vi "MSTAutoSummarySpecial.vi"() -> ()   [LabVIEW 2012]
uses:
  <vilib>/Utility/NIReport.llb/NI_report.lvclass
  <vilib>/addons/database/Connection.llb/DB Tools Open Connec (Path).vi
  <vilib>/addons/database/Connection.llb/Conn Execute.vi
  <vilib>/addons/database/Recordset.llb/Rec Fetch Recordset Data (R).vi
  <vilib>/addons/database/Recordset.llb/Rec Destroy - Connection.vi
  <vilib>/Utility/NIReport.llb/Append Text Table to Report (wrap).vi
  <vilib>/addons/database/_DB Variant To Data/Database Variant To Data.xnode
  <vilib>/addons/database/NI_Database_API.lvlib
  <vilib>/Utility/NIReport.llb/Excel/NI_Excel.lvclass
  <vilib>/addons/_office/NI_ReportGenerationToolkit.lvlib
panel:
  in  "Report Template":path=path "O:/Monitor/Report/MSTDailyReport.xls"
  in  "Table Control":string[][](table)
  in  "Table Control 2":string[][](table)
  out "error out 4":errorcluster
  out "error out 3":errorcluster
  out "appended array 3":string[](array[string])
  out "recordset data 3":variant[][](array[variant])
  out "error out":errorcluster
  out "appended array":string[](array[string])
  out "recordset data":variant[][](array[variant])
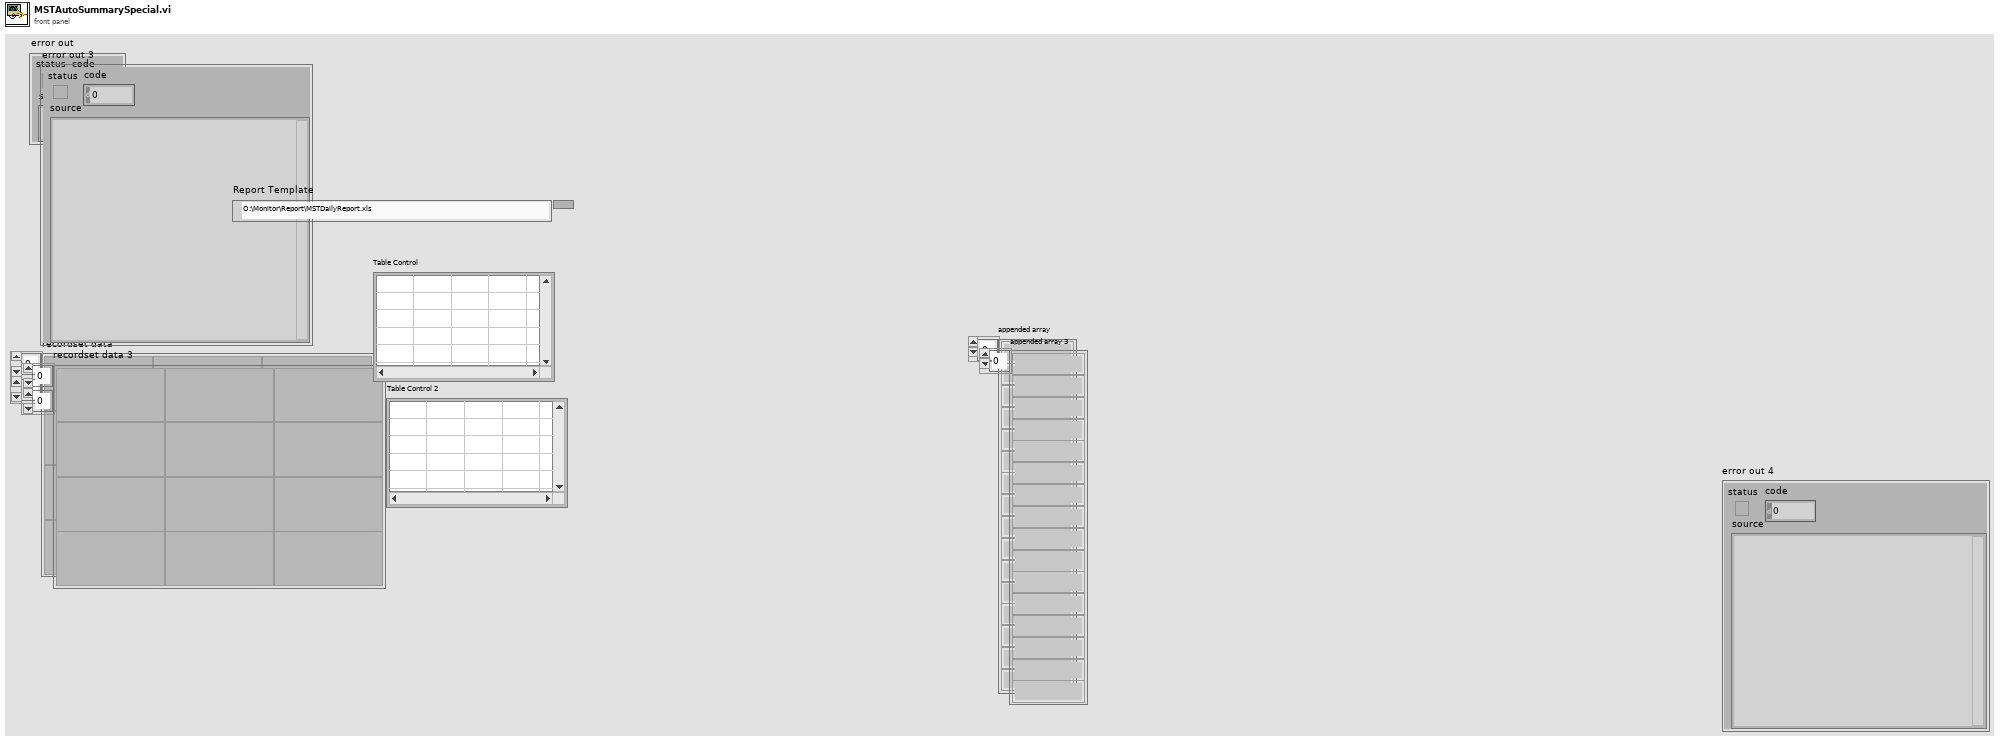
[diagram p1: front panel]
types:
  T1 = typedef "NI_Database_API.lvlib/Conn ObjectReference.ctl" = refnum<k1>
  T2 = typedef "NI_Database_API.lvlib/Rec ObjectReference.ctl" = refnum<k1>
  T3 = enum16{"Standard Report", "HTML", "Word", "Excel"}
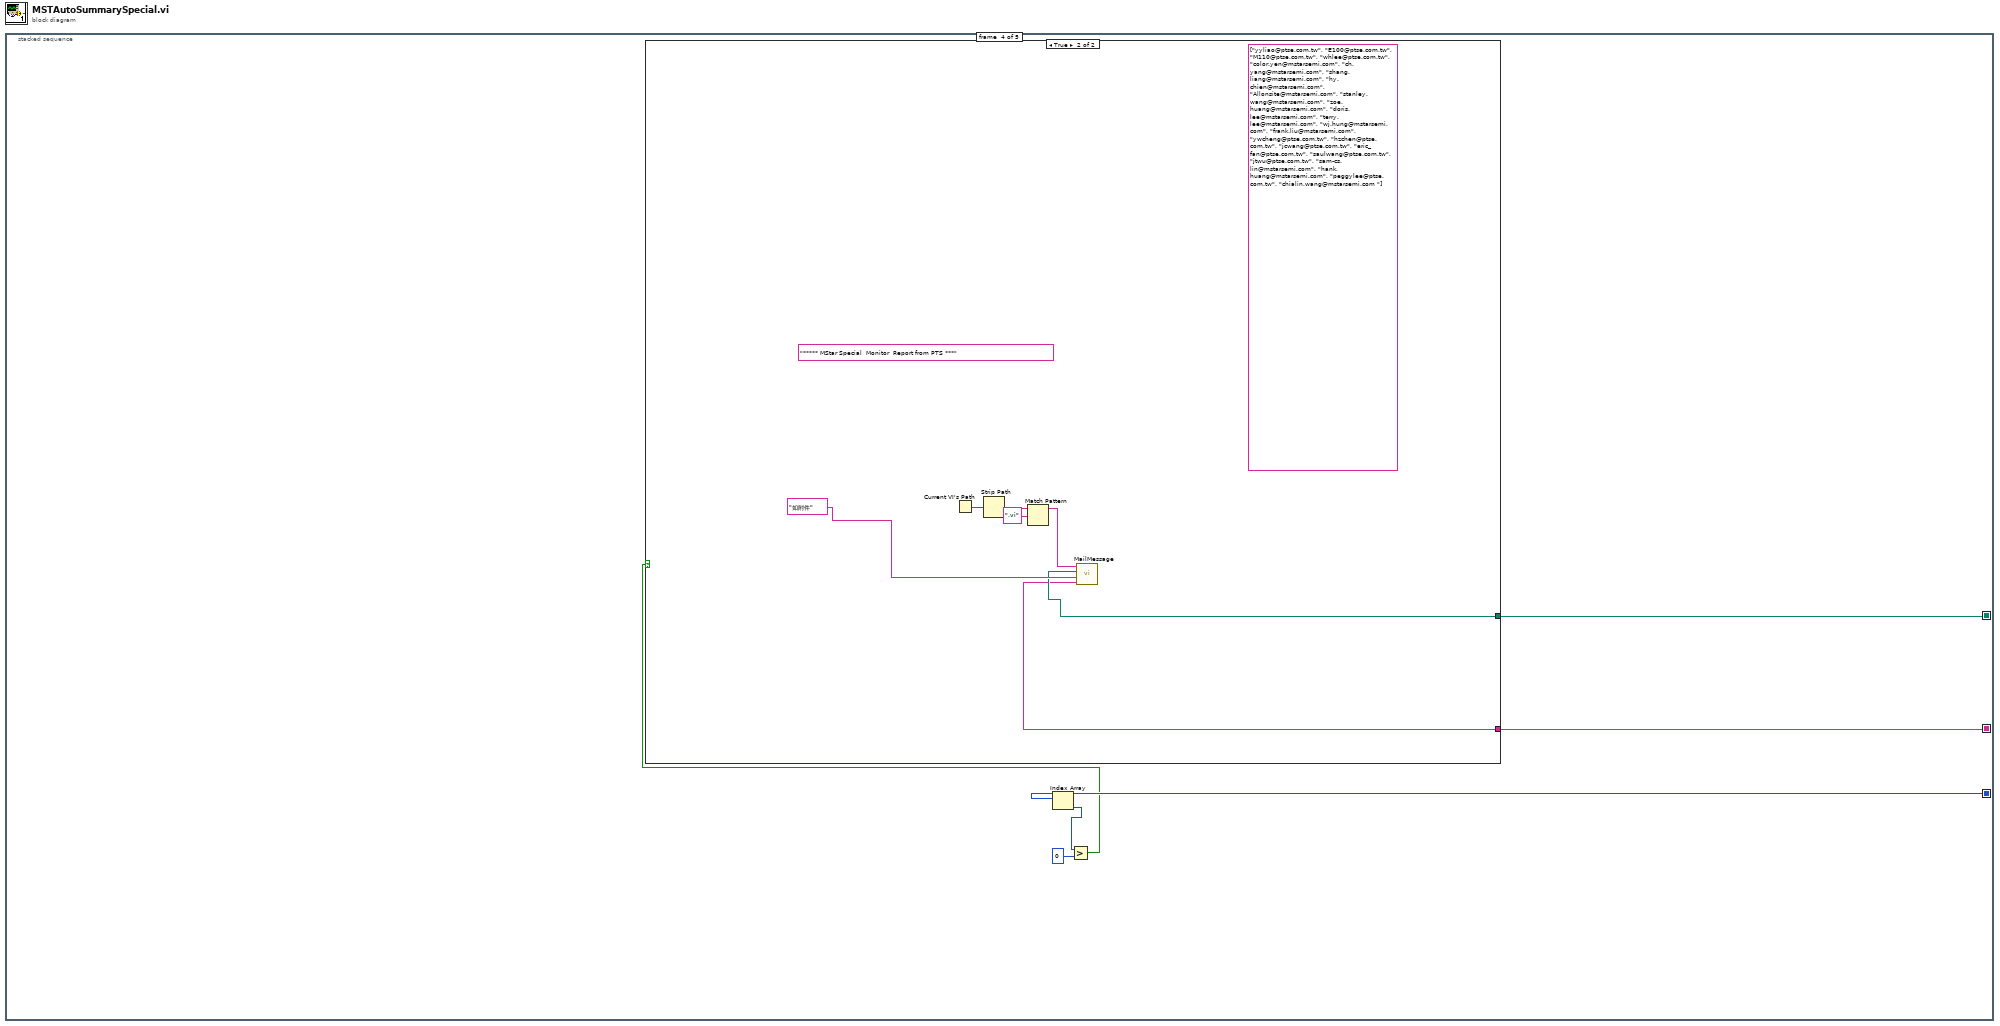
[diagram p0: block diagram]
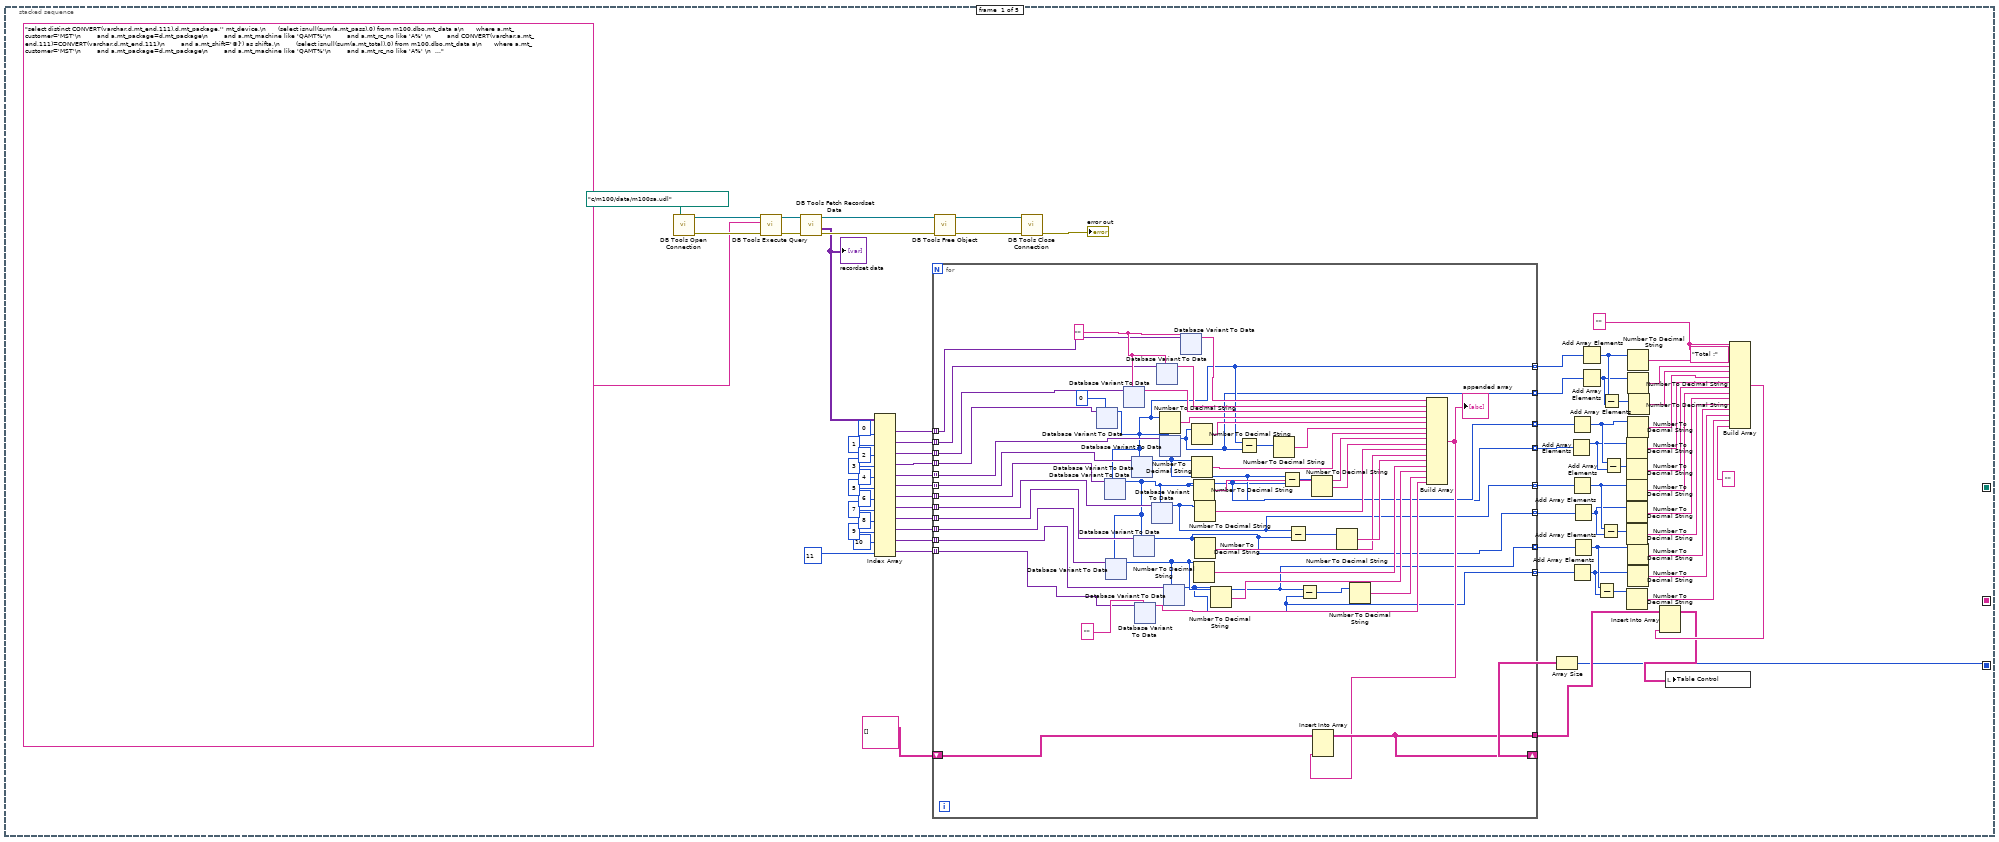
[diagram p2: hidden frame]
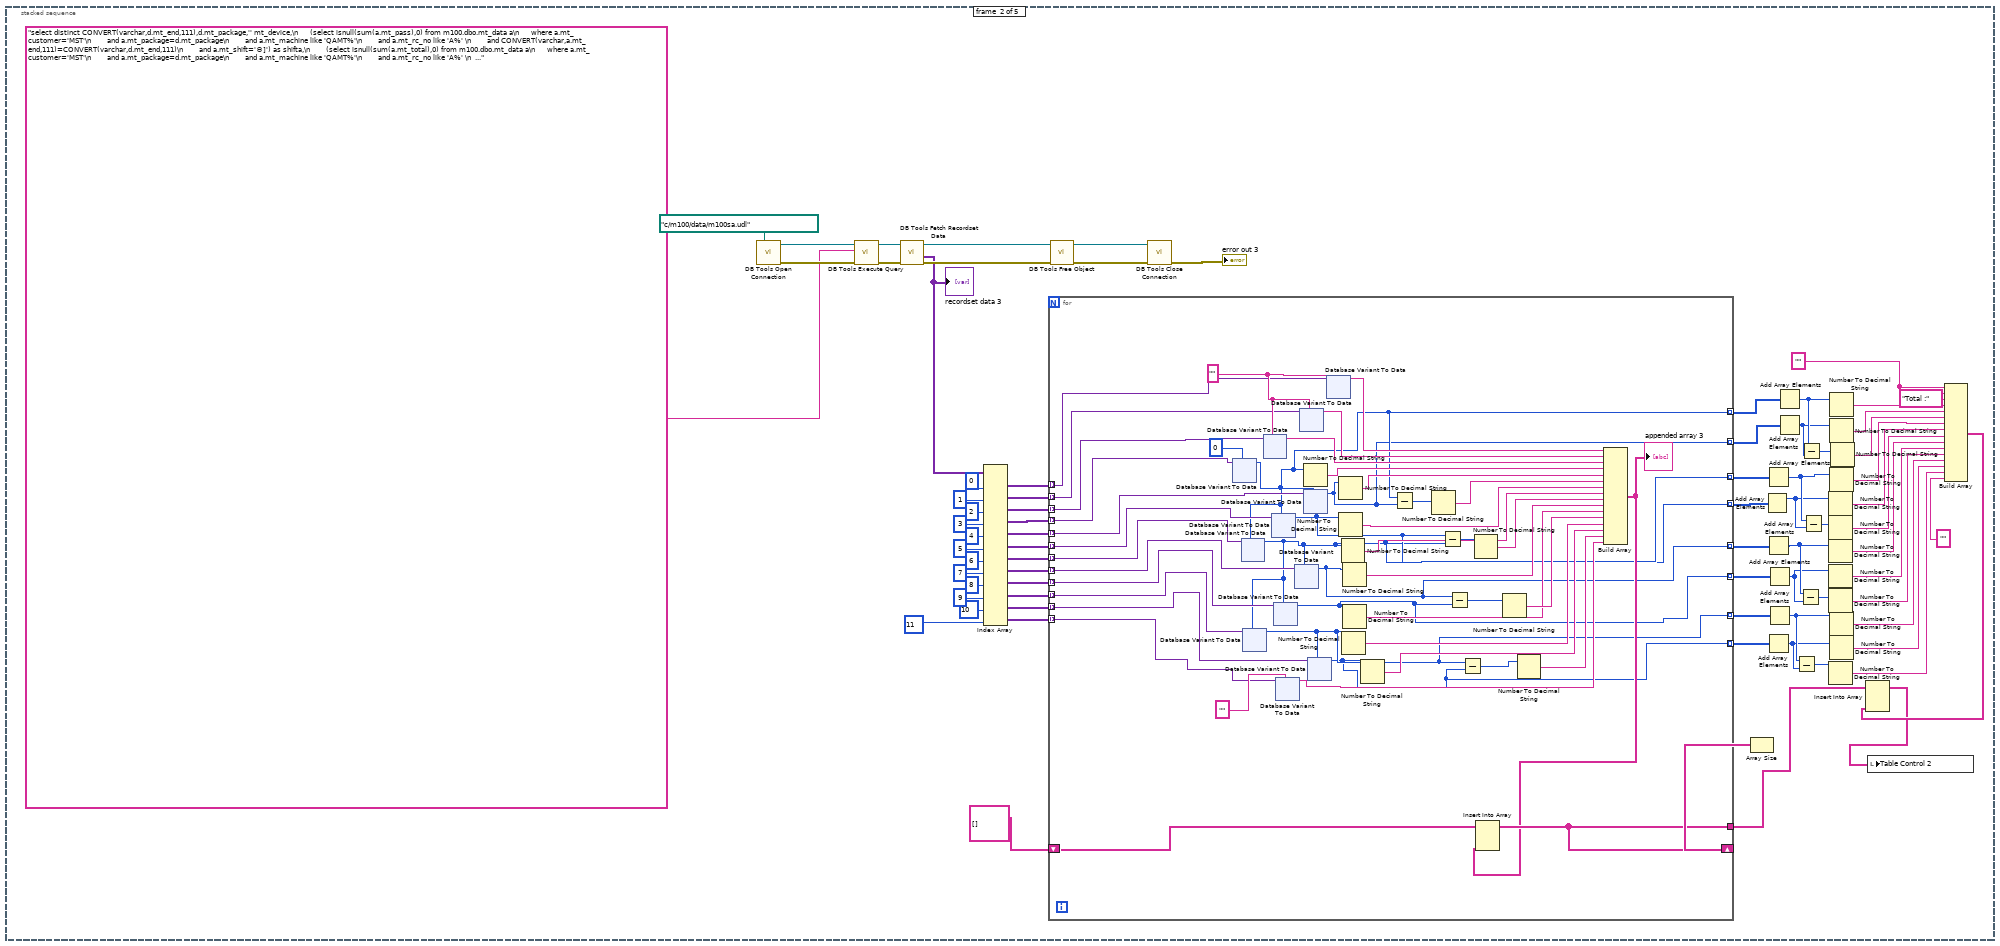
[diagram p3: hidden frame]
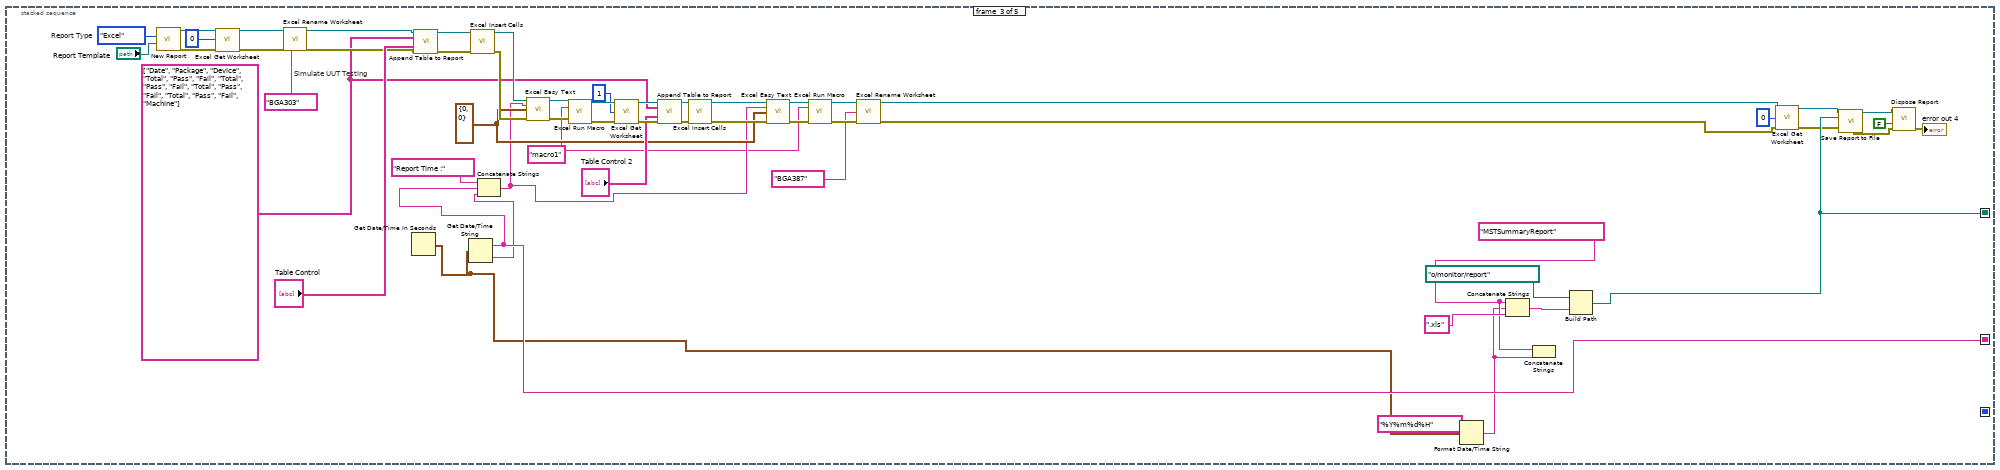
[diagram p4: hidden frame]
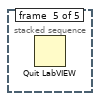
[diagram p6: hidden frame]
diagram:
  n1 = stacked-sequence {
    seq-local: [_ _ w1055 _ _] -> [_ _ _ w1075 _]
    seq-local: [_ _ w1054 _ _] -> [_ _ _ w1074 _]
    seq-local: [w1 _ _ _ _] -> [_ _ _ w1073 _]
    frame #0 {
      w37 = ""
      n2 = call-poly <vilib>:"DB Tools Open Connection.vi"("connection information"=path "c:/m100/data/m100sa.udl") -> ("error out"=w72:errorcluster, "connection reference"=w76:T1)  [unwired: 7 in]
      n3 = call-poly <vilib>:"DB Tools Execute Query.vi"("error in (no error)"=w72, "SQL query"="select distinct CONVERT(varchar,d.mt_end,111),d.mt_package,'' mt_device,\n      (select isnull(sum(a.mt_pass),0) from m100.dbo.mt_data a\n      where a.mt_customer='MST'\n        and a.mt_package=d.mt_package\n        and a.mt_machine like 'QAMT%'\n        and a.mt_rc_no like 'A%' \n        and CONVERT(varchar,a.mt_end,111)=CONVERT(varchar,d.mt_end,111)\n        and a.mt_shift='©]') as shifta,\n        (select isnull(sum(a.mt_total),0) from m100.dbo.mt_data a\n      where a.mt_customer='MST'\n        and a.mt_package=d.mt_package\n        and a.mt_machine like 'QAMT%'\n        and a.mt_rc_no like 'A%' \n        and CONVERT(varchar,a.mt_end,111)=CONVERT(varchar,d.mt_end,111)\n        and a.mt_shift='©]') as shifta1,\n        (select isnull(sum(b.mt_pass),0) from m100.dbo.mt_data b\n      where b.mt_customer='MST'\n        and b.mt_package=d.mt_package\n        and b.mt_machine like 'QAMT%'\n        and b.mt_rc_no like 'A%' \n        and CONVERT(varchar,b.mt_end,111)=CONVERT(varchar,d.mt_end,111)\n        and b.mt_shift='¦­') as shiftb,\n        (select isnull(sum(b.mt_total),0) from m100.dbo.mt_data b\n      where b.mt_customer='MST'\n        and b.mt_package=d.mt_package\n        and b.mt_machine like 'QAMT%'\n        and b.mt_rc_no like 'A%' \n        and CONVERT(varchar,b.mt_end,111)=CONVERT(varchar,d.mt_end,111)\n        and b.mt_shift='¦­') as shiftb1,\n        (select isnull(sum(c.mt_pass),0) from m100.dbo.mt_data c\n      where c.mt_customer='MST'\n        and c.mt_package=d.mt_package\n        and c.mt_machine like 'QAMT%'\n        and c.mt_rc_no like 'A%' \n        and CONVERT(varchar,c.mt_end,111)=CONVERT(varchar,d.mt_end,111)\n        and c.mt_shift='¤¤') as shiftc,\n        (select isnull(sum(c.mt_total),0) from m100.dbo.mt_data c\n      where c.mt_customer='MST'\n        and c.mt_package=d.mt_package\n        and c.mt_machine like 'QAMT%'\n        and c.mt_rc_no like 'A%' \n        and CONVERT(varchar,c.mt_end,111)=CONVERT(varchar,d.mt_end,111)\n        and c.mt_shift='¤¤') as shiftc1,\n        SUM(mt_pass),SUM(mt_total),master.dbo.GetEntityNameFromDateToDateByPackage('MST',d.mt_package,CONVERT(varchar,d.mt_end,111),CONVERT(varchar,d.mt_end,111))\n  FROM [m100].[dbo].[mt_data] d\n  WHERE d.mt_customer='MST'\n    and d.mt_machine like 'QAMT%'\n    and d.mt_package like '%BGA303%'\n    AND CONVERT(varchar,d.mt_end,111) >= convert(varchar,getdate()-30,111)\n    AND CONVERT(varchar,d.mt_end,111) >= '2016/03/30'\n    and d.mt_pass > 0 and d.mt_rc_no like 'A%'\n      group by CONVERT(varchar,d.mt_end,111),d.mt_package", "connection reference"=w76) -> ("error out"=w71:errorcluster, "recordset reference"=w75:T2)  [unwired: 5 in]
      n4 = call-poly <vilib>:"DB Tools Fetch Recordset Data.vi"("error in (no error)"=w71, "recordset reference"=w75) -> ("error out"=w70:errorcluster, "recordset data"=w40:variant[][], "recordset reference out"=w74:T2)  [unwired: 3 in]
      "recordset data" <- w40
      n5 = Index Array(array=w40, index (col) #1=0 ("index (row)"), index (col) #2=1 ("index (col)"), index (col) #3=2 ("disabled index (col)"), index (col) #4=3 ("index (col)"), index (col) #5=4 ("index (col)"), index (col) #6=5 ("index (col)"), index (col) #7=6 ("index (col)"), index (col) #8=7 ("index (col)"), index (col) #9=8 ("index (col)"), index (col) #10=9 ("index (col)"), index (col) #11=10 ("index (col)"), index (col) #12=11 ("index (col)")) -> (element #1=w44:variant[], element #2=w43:variant[], element #3=w57:variant[], element #4=w56:variant[], element #5=w55:variant[], element #6=w54:variant[], element #7=w53:variant[], element #8=w52:variant[], element #9=w51:variant[], element #10=w50:variant[], element #11=w49:variant[], element #12=w48:variant[])  [unwired: 12 in]
      n6 = for {
        tunnel: w57 -> [w96] mode=indexing
        tunnel: w56 -> [w95] mode=indexing
        tunnel: w55 -> [w94] mode=indexing
        tunnel: w54 -> [w93] mode=indexing
        tunnel: w53 -> [w92] mode=indexing
        tunnel: w52 -> [w91] mode=indexing
        tunnel: w51 -> [w90] mode=indexing
        tunnel: w50 -> [w89] mode=indexing
        tunnel: w49 -> [w88] mode=indexing
        tunnel: w48 -> [w87] mode=indexing
        tunnel: [w123] -> w30
        shift-right: [w123] -> w46
        shift-left: string[][] [] ("array") -> [w122]
        tunnel: w44 -> [w98] mode=indexing
        tunnel: w43 -> [w97] mode=indexing
        tunnel: [w85] -> w39 mode=indexing
        tunnel: [w84] -> w38 mode=indexing
        tunnel: [w83] -> w28 mode=indexing
        tunnel: [w82] -> w27 mode=indexing
        tunnel: [w81] -> w18 mode=indexing
        tunnel: [w80] -> w17 mode=indexing
        tunnel: [w79] -> w10 mode=indexing
        tunnel: [w78] -> w9 mode=indexing
        w121 = ""
        n7 = xnode "Database Variant To Data"("database variant"=w95, "type"=0) -> ("data"=w85:i32)  [unwired: 1 in, 1 out]
        n8 = xnode "Database Variant To Data"("database variant"=w92, "type"=w85) -> ("data"=w82:i32)  [unwired: 1 in, 1 out]
        n9 = xnode "Database Variant To Data"("database variant"=w89, "type"=w82) -> ("data"=w79:i32)  [unwired: 1 in, 1 out]
        n10 = xnode "Database Variant To Data"("database variant"=w96, "type"=w121) -> ("data"=w104:string)  [unwired: 1 in, 1 out]
        n11 = xnode "Database Variant To Data"("database variant"=w93, "type"=w85) -> ("data"=w83:i32)  [unwired: 1 in, 1 out]
        n12 = xnode "Database Variant To Data"("database variant"=w90, "type"=w82) -> ("data"=w80:i32)  [unwired: 1 in, 1 out]
        n13 = xnode "Database Variant To Data"("database variant"=w87, "type"="") -> ("data"=w116:string)  [unwired: 1 in, 1 out]
        n14 = xnode "Database Variant To Data"("database variant"=w91, "type"=w82) -> ("data"=w81:i32)  [unwired: 1 in, 1 out]
        n15 = xnode "Database Variant To Data"("database variant"=w97, "type"=w121) -> ("data"=w101:string)  [unwired: 1 in, 1 out]
        n16 = Number To Decimal String(number=w85) -> (decimal integer string=w103:string)  [unwired: 1 in]
        n17 = xnode "Database Variant To Data"("database variant"=w94, "type"=w85) -> ("data"=w84:i32)  [unwired: 1 in, 1 out]
        n18 = xnode "Database Variant To Data"("database variant"=w88, "type"=w79) -> ("data"=w78:i32)  [unwired: 1 in, 1 out]
        n19 = xnode "Database Variant To Data"("database variant"=w98, "type"=w121) -> ("data"=w105:string)  [unwired: 1 in, 1 out]
        n20 = Number To Decimal String(number=w84) -> (decimal integer string=w102:string)  [unwired: 1 in]
        n21 = Number To Decimal String(number=w83) -> (decimal integer string=w119:string)  [unwired: 1 in]
        n22 = Number To Decimal String(number=w82) -> (decimal integer string=w118:string)  [unwired: 1 in]
        n23 = Number To Decimal String(number=w79) -> (decimal integer string=w112:string)  [unwired: 1 in]
        n24 = Number To Decimal String(number=w81) -> (decimal integer string=w108:string)  [unwired: 1 in]
        n25 = Number To Decimal String(number=w80) -> (decimal integer string=w109:string)  [unwired: 1 in]
        n26 = Number To Decimal String(number=w78) -> (decimal integer string=w113:string)  [unwired: 1 in]
        n27 = Subtract(x=w85, y=w84) -> (x-y=w100:i32)
        n28 = Number To Decimal String(number=w100) -> (decimal integer string=w99:string)  [unwired: 1 in]
        n29 = Subtract(x=w83, y=w82) -> (x-y=w107:i32)
        n30 = Subtract(x=w81, y=w80) -> (x-y=w111:i32)
        n31 = Subtract(x=w79, y=w78) -> (x-y=w115:i32)
        n32 = Number To Decimal String(number=w107) -> (decimal integer string=w106:string)  [unwired: 1 in]
        n33 = Number To Decimal String(number=w111) -> (decimal integer string=w110:string)  [unwired: 1 in]
        n34 = Number To Decimal String(number=w115) -> (decimal integer string=w114:string)  [unwired: 1 in]
        n35 = Build Array(w105, w101, w104, w103, w102, w99, w119, w118, w106, w108, w109, w110, w112, w113, w114, w116) -> (w86:string[])
        "appended array" <- w86
        n36 = Insert Into Array(array=w122, new element=w86) -> (w123:string[][])  [unwired: 2 in]
      }
      n37 = call-poly <vilib>:"DB Tools Free Object.vi"("error in (no error)"=w70, "recordset reference"=w74) -> ("error out"=w69:errorcluster, "connection reference"=w73:T1)  [unwired: 8 in]
      n38 = call <vilib>:"DB Tools Close Connection.vi"("error in (no error)"=w69, "connection reference"=w73) -> ("error out"=→"error out":errorcluster)  [unwired: 5 in]
      n39 = Array Size(array=w46) -> (size(s)=w1:i32[])
      n40 = Add Array Elements(numeric array=w27) -> (sum=w21:i32)
      n41 = Add Array Elements(numeric array=w28) -> (sum=w22:i32)
      n42 = Add Array Elements(numeric array=w18) -> (sum=w14:i32)
      n43 = Add Array Elements(numeric array=w9) -> (sum=w7:i32)
      n44 = Add Array Elements(numeric array=w17) -> (sum=w13:i32)
      n45 = Add Array Elements(numeric array=w10) -> (sum=w8:i32)
      n46 = Add Array Elements(numeric array=w39) -> (sum=w34:i32)
      n47 = Add Array Elements(numeric array=w38) -> (sum=w33:i32)
      n48 = Subtract(x=w8, y=w7) -> (x-y=w6:i32)
      n49 = Subtract(x=w14, y=w13) -> (x-y=w11:i32)
      n50 = Subtract(x=w34, y=w33) -> (x-y=w26:i32)
      n51 = Subtract(x=w22, y=w21) -> (x-y=w19:i32)
      n52 = Number To Decimal String(number=w21) -> (decimal integer string=w23:string)  [unwired: 1 in]
      n53 = Number To Decimal String(number=w19) -> (decimal integer string=w20:string)  [unwired: 1 in]
      n54 = Number To Decimal String(number=w14) -> (decimal integer string=w16:string)  [unwired: 1 in]
      n55 = Number To Decimal String(number=w13) -> (decimal integer string=w15:string)  [unwired: 1 in]
      n56 = Number To Decimal String(number=w11) -> (decimal integer string=w12:string)  [unwired: 1 in]
      n57 = Number To Decimal String(number=w6) -> (decimal integer string=w3:string)  [unwired: 1 in]
      n58 = Number To Decimal String(number=w34) -> (decimal integer string=w36:string)  [unwired: 1 in]
      n59 = Number To Decimal String(number=w33) -> (decimal integer string=w35:string)  [unwired: 1 in]
      n60 = Number To Decimal String(number=w22) -> (decimal integer string=w25:string)  [unwired: 1 in]
      n61 = Number To Decimal String(number=w8) -> (decimal integer string=w5:string)  [unwired: 1 in]
      n62 = Number To Decimal String(number=w7) -> (decimal integer string=w4:string)  [unwired: 1 in]
      n63 = Number To Decimal String(number=w26) -> (decimal integer string=w32:string)  [unwired: 1 in]
      n64 = Build Array(w37, w37, "Total :" ("element"), w36, w35, w32, w25, w23, w20, w16, w15, w12, w5, w4, w3, "") -> (w31:string[])
      n65 = Insert Into Array(array=w30, new element=w31) -> (w29:string[][])  [unwired: 2 in]
      n66 = local write "Table Control"(w29) -> ()
    }
    frame #1 {
      w543 = ""
      n67 = call-poly <vilib>:"DB Tools Open Connection.vi"("connection information"=path "c:/m100/data/m100sa.udl") -> ("error out"=w578:errorcluster, "connection reference"=w582:T1)  [unwired: 7 in]
      n68 = call-poly <vilib>:"DB Tools Execute Query.vi"("error in (no error)"=w578, "SQL query"="select distinct CONVERT(varchar,d.mt_end,111),d.mt_package,'' mt_device,\n      (select isnull(sum(a.mt_pass),0) from m100.dbo.mt_data a\n      where a.mt_customer='MST'\n        and a.mt_package=d.mt_package\n        and a.mt_machine like 'QAMT%'\n        and a.mt_rc_no like 'A%' \n        and CONVERT(varchar,a.mt_end,111)=CONVERT(varchar,d.mt_end,111)\n        and a.mt_shift='©]') as shifta,\n        (select isnull(sum(a.mt_total),0) from m100.dbo.mt_data a\n      where a.mt_customer='MST'\n        and a.mt_package=d.mt_package\n        and a.mt_machine like 'QAMT%'\n        and a.mt_rc_no like 'A%' \n        and CONVERT(varchar,a.mt_end,111)=CONVERT(varchar,d.mt_end,111)\n        and a.mt_shift='©]') as shifta1,\n        (select isnull(sum(b.mt_pass),0) from m100.dbo.mt_data b\n      where b.mt_customer='MST'\n        and b.mt_package=d.mt_package\n        and b.mt_machine like 'QAMT%'\n        and b.mt_rc_no like 'A%' \n        and CONVERT(varchar,b.mt_end,111)=CONVERT(varchar,d.mt_end,111)\n        and b.mt_shift='¦­') as shiftb,\n        (select isnull(sum(b.mt_total),0) from m100.dbo.mt_data b\n      where b.mt_customer='MST'\n        and b.mt_package=d.mt_package\n        and b.mt_machine like 'QAMT%'\n        and b.mt_rc_no like 'A%' \n        and CONVERT(varchar,b.mt_end,111)=CONVERT(varchar,d.mt_end,111)\n        and b.mt_shift='¦­') as shiftb1,\n        (select isnull(sum(c.mt_pass),0) from m100.dbo.mt_data c\n      where c.mt_customer='MST'\n        and c.mt_package=d.mt_package\n        and c.mt_machine like 'QAMT%'\n        and c.mt_rc_no like 'A%' \n        and CONVERT(varchar,c.mt_end,111)=CONVERT(varchar,d.mt_end,111)\n        and c.mt_shift='¤¤') as shiftc,\n        (select isnull(sum(c.mt_total),0) from m100.dbo.mt_data c\n      where c.mt_customer='MST'\n        and c.mt_package=d.mt_package\n        and c.mt_machine like 'QAMT%'\n        and c.mt_rc_no like 'A%' \n        and CONVERT(varchar,c.mt_end,111)=CONVERT(varchar,d.mt_end,111)\n        and c.mt_shift='¤¤') as shiftc1,\n        SUM(mt_pass),SUM(mt_total),master.dbo.GetEntityNameFromDateToDateByPackage('MST',d.mt_package,CONVERT(varchar,d.mt_end,111),CONVERT(varchar,d.mt_end,111))\n  FROM [m100].[dbo].[mt_data] d\n  WHERE d.mt_customer='MST'\n    and d.mt_machine like 'QAMT%'\n    and d.mt_package like '%BGA387%'\n    AND CONVERT(varchar,d.mt_end,111) >= convert(varchar,getdate()-30,111)\n    AND CONVERT(varchar,d.mt_end,111) >= '2016/03/30'\n    and d.mt_pass > 0 and d.mt_rc_no like 'A%'\n      group by CONVERT(varchar,d.mt_end,111),d.mt_package", "connection reference"=w582) -> ("error out"=w577:errorcluster, "recordset reference"=w581:T2)  [unwired: 5 in]
      n69 = call-poly <vilib>:"DB Tools Fetch Recordset Data.vi"("error in (no error)"=w577, "recordset reference"=w581) -> ("error out"=w576:errorcluster, "recordset data"=w546:variant[][], "recordset reference out"=w580:T2)  [unwired: 3 in]
      "recordset data 3" <- w546
      n70 = Index Array(array=w546, index (col) #1=0 ("index (row)"), index (col) #2=1 ("index (col)"), index (col) #3=2 ("disabled index (col)"), index (col) #4=3 ("index (col)"), index (col) #5=4 ("index (col)"), index (col) #6=5 ("index (col)"), index (col) #7=6 ("index (col)"), index (col) #8=7 ("index (col)"), index (col) #9=8 ("index (col)"), index (col) #10=9 ("index (col)"), index (col) #11=10 ("index (col)"), index (col) #12=11 ("index (col)")) -> (element #1=w550:variant[], element #2=w549:variant[], element #3=w563:variant[], element #4=w562:variant[], element #5=w561:variant[], element #6=w560:variant[], element #7=w559:variant[], element #8=w558:variant[], element #9=w557:variant[], element #10=w556:variant[], element #11=w555:variant[], element #12=w554:variant[])  [unwired: 12 in]
      n71 = for {
        tunnel: w563 -> [w602] mode=indexing
        tunnel: w562 -> [w601] mode=indexing
        tunnel: w561 -> [w600] mode=indexing
        tunnel: w560 -> [w599] mode=indexing
        tunnel: w559 -> [w598] mode=indexing
        tunnel: w558 -> [w597] mode=indexing
        tunnel: w557 -> [w596] mode=indexing
        tunnel: w556 -> [w595] mode=indexing
        tunnel: w555 -> [w594] mode=indexing
        tunnel: w554 -> [w593] mode=indexing
        tunnel: [w629] -> w536
        shift-right: [w629] -> w552
        shift-left: string[][] [] ("array") -> [w628]
        tunnel: w550 -> [w604] mode=indexing
        tunnel: w549 -> [w603] mode=indexing
        tunnel: [w591] -> w545 mode=indexing
        tunnel: [w590] -> w544 mode=indexing
        tunnel: [w589] -> w534 mode=indexing
        tunnel: [w588] -> w533 mode=indexing
        tunnel: [w587] -> w524 mode=indexing
        tunnel: [w586] -> w523 mode=indexing
        tunnel: [w585] -> w516 mode=indexing
        tunnel: [w584] -> w515 mode=indexing
        w627 = ""
        n72 = xnode "Database Variant To Data"("database variant"=w601, "type"=0) -> ("data"=w591:i32)  [unwired: 1 in, 1 out]
        n73 = xnode "Database Variant To Data"("database variant"=w598, "type"=w591) -> ("data"=w588:i32)  [unwired: 1 in, 1 out]
        n74 = xnode "Database Variant To Data"("database variant"=w595, "type"=w588) -> ("data"=w585:i32)  [unwired: 1 in, 1 out]
        n75 = xnode "Database Variant To Data"("database variant"=w602, "type"=w627) -> ("data"=w610:string)  [unwired: 1 in, 1 out]
        n76 = xnode "Database Variant To Data"("database variant"=w599, "type"=w591) -> ("data"=w589:i32)  [unwired: 1 in, 1 out]
        n77 = xnode "Database Variant To Data"("database variant"=w596, "type"=w588) -> ("data"=w586:i32)  [unwired: 1 in, 1 out]
        n78 = xnode "Database Variant To Data"("database variant"=w593, "type"="") -> ("data"=w622:string)  [unwired: 1 in, 1 out]
        n79 = xnode "Database Variant To Data"("database variant"=w597, "type"=w588) -> ("data"=w587:i32)  [unwired: 1 in, 1 out]
        n80 = xnode "Database Variant To Data"("database variant"=w603, "type"=w627) -> ("data"=w607:string)  [unwired: 1 in, 1 out]
        n81 = Number To Decimal String(number=w591) -> (decimal integer string=w609:string)  [unwired: 1 in]
        n82 = xnode "Database Variant To Data"("database variant"=w600, "type"=w591) -> ("data"=w590:i32)  [unwired: 1 in, 1 out]
        n83 = xnode "Database Variant To Data"("database variant"=w594, "type"=w585) -> ("data"=w584:i32)  [unwired: 1 in, 1 out]
        n84 = xnode "Database Variant To Data"("database variant"=w604, "type"=w627) -> ("data"=w611:string)  [unwired: 1 in, 1 out]
        n85 = Number To Decimal String(number=w590) -> (decimal integer string=w608:string)  [unwired: 1 in]
        n86 = Number To Decimal String(number=w589) -> (decimal integer string=w625:string)  [unwired: 1 in]
        n87 = Number To Decimal String(number=w588) -> (decimal integer string=w624:string)  [unwired: 1 in]
        n88 = Number To Decimal String(number=w585) -> (decimal integer string=w618:string)  [unwired: 1 in]
        n89 = Number To Decimal String(number=w587) -> (decimal integer string=w614:string)  [unwired: 1 in]
        n90 = Number To Decimal String(number=w586) -> (decimal integer string=w615:string)  [unwired: 1 in]
        n91 = Number To Decimal String(number=w584) -> (decimal integer string=w619:string)  [unwired: 1 in]
        n92 = Subtract(x=w591, y=w590) -> (x-y=w606:i32)
        n93 = Number To Decimal String(number=w606) -> (decimal integer string=w605:string)  [unwired: 1 in]
        n94 = Subtract(x=w589, y=w588) -> (x-y=w613:i32)
        n95 = Subtract(x=w587, y=w586) -> (x-y=w617:i32)
        n96 = Subtract(x=w585, y=w584) -> (x-y=w621:i32)
        n97 = Number To Decimal String(number=w613) -> (decimal integer string=w612:string)  [unwired: 1 in]
        n98 = Number To Decimal String(number=w617) -> (decimal integer string=w616:string)  [unwired: 1 in]
        n99 = Number To Decimal String(number=w621) -> (decimal integer string=w620:string)  [unwired: 1 in]
        n100 = Build Array(w611, w607, w610, w609, w608, w605, w625, w624, w612, w614, w615, w616, w618, w619, w620, w622) -> (w592:string[])
        "appended array 3" <- w592
        n101 = Insert Into Array(array=w628, new element=w592) -> (w629:string[][])  [unwired: 2 in]
      }
      n102 = call-poly <vilib>:"DB Tools Free Object.vi"("error in (no error)"=w576, "recordset reference"=w580) -> ("error out"=w575:errorcluster, "connection reference"=w579:T1)  [unwired: 8 in]
      n103 = call <vilib>:"DB Tools Close Connection.vi"("error in (no error)"=w575, "connection reference"=w579) -> ("error out"=→"error out 3":errorcluster)  [unwired: 5 in]
      n104 = Array Size(array=w552) -> ()  [unwired: 1 out]
      n105 = Add Array Elements(numeric array=w533) -> (sum=w527:i32)
      n106 = Add Array Elements(numeric array=w534) -> (sum=w528:i32)
      n107 = Add Array Elements(numeric array=w524) -> (sum=w520:i32)
      n108 = Add Array Elements(numeric array=w515) -> (sum=w513:i32)
      n109 = Add Array Elements(numeric array=w523) -> (sum=w519:i32)
      n110 = Add Array Elements(numeric array=w516) -> (sum=w514:i32)
      n111 = Add Array Elements(numeric array=w545) -> (sum=w540:i32)
      n112 = Add Array Elements(numeric array=w544) -> (sum=w539:i32)
      n113 = Subtract(x=w514, y=w513) -> (x-y=w512:i32)
      n114 = Subtract(x=w520, y=w519) -> (x-y=w517:i32)
      n115 = Subtract(x=w540, y=w539) -> (x-y=w532:i32)
      n116 = Subtract(x=w528, y=w527) -> (x-y=w525:i32)
      n117 = Number To Decimal String(number=w527) -> (decimal integer string=w529:string)  [unwired: 1 in]
      n118 = Number To Decimal String(number=w525) -> (decimal integer string=w526:string)  [unwired: 1 in]
      n119 = Number To Decimal String(number=w520) -> (decimal integer string=w522:string)  [unwired: 1 in]
      n120 = Number To Decimal String(number=w519) -> (decimal integer string=w521:string)  [unwired: 1 in]
      n121 = Number To Decimal String(number=w517) -> (decimal integer string=w518:string)  [unwired: 1 in]
      n122 = Number To Decimal String(number=w512) -> (decimal integer string=w509:string)  [unwired: 1 in]
      n123 = Number To Decimal String(number=w540) -> (decimal integer string=w542:string)  [unwired: 1 in]
      n124 = Number To Decimal String(number=w539) -> (decimal integer string=w541:string)  [unwired: 1 in]
      n125 = Number To Decimal String(number=w528) -> (decimal integer string=w531:string)  [unwired: 1 in]
      n126 = Number To Decimal String(number=w514) -> (decimal integer string=w511:string)  [unwired: 1 in]
      n127 = Number To Decimal String(number=w513) -> (decimal integer string=w510:string)  [unwired: 1 in]
      n128 = Number To Decimal String(number=w532) -> (decimal integer string=w538:string)  [unwired: 1 in]
      n129 = Build Array(w543, w543, "Total :" ("element"), w542, w541, w538, w531, w529, w526, w522, w521, w518, w511, w510, w509, "") -> (w537:string[])
      n130 = Insert Into Array(array=w536, new element=w537) -> (w535:string[][])  [unwired: 2 in]
      n131 = local write "Table Control 2"(w535) -> ()
    }
    frame #2 {
      w1016 = "macro1" ("macro name")
      w1056 = "MSTSummaryReport"
      w1019 = string[] ["Date", "Package", "Device", "Total", "Pass", "Fail", "Total", "Pass", "Fail", "Total", "Pass", "Fail", "Total", "Pass", "Fail", "Machine"] ("row headers")
      w1018 = cluster{"row":i32, "column":i32} {"row"=0, "column"=0} ("end (-1, -1)")
      w1069 = T3."Excel"  # Report Type
      # "Simulate UUT Testing"
      n132 = call <vilib>:"New Report.vi"("report type"=w1069, "template (empty)"="Report Template") -> ("report out"=w1065:refnum<class "NI_report.lvclass">, "error out"=w1064:errorcluster)  [unwired: 12 in]
      n133 = call <vilib>:"Excel Get Worksheet.vi"("report in"=w1065, "worksheet index (0)"=0, "error in (no error)"=w1064) -> ("report out"=w1032:refnum<class "NI_report.lvclass">, "error out"=w1031:errorcluster)  [unwired: 11 in]
      n134 = call <vilib>:"Excel Rename Worksheet.vi"("report in"=w1032, "worksheet name (\"\")"="BGA303" ("worksheet name (\"\")"), "error in (no error)"=w1031) -> ("report out"=w1030:refnum<class "NI_report.lvclass">, "error out"=w1029:errorcluster)  [unwired: 11 in]
      n135 = Get Date/Time In Seconds() -> (seconds since 1Jan1904=w1022:timestamp)
      n136 = call-poly <vilib>:"Append Table to Report.vi"("report in"=w1030, "column headers"=w1019, "text data"="Table Control", "error in (no error)"=w1029) -> ("report out"=w1067:refnum<class "NI_report.lvclass">, "error out"=w1066:errorcluster)  [unwired: 8 in, 2 out]
      n137 = Get Date/Time String(seconds (now)=w1022) -> (date string=w1054:string, time string=w1025:string)  [unwired: 2 in]
      n138 = call <vilib>:"Excel Insert Cells.vi"("report in"=w1067, "error in (no error)"=w1066) -> ("report out"=w1063:refnum<class "NI_report.lvclass">, "error out"=w1062:errorcluster)  [unwired: 12 in]
      n139 = Concatenate Strings("Report Time :" ("string"), w1054, w1025) -> (w1017:string)
      n140 = call <vilib>:"Excel Easy Text.vi"("report in"=w1063, "text"=w1017, "start (-1, -1)"=w1018, "error in (no error)"=w1062) -> ("report out"=w1052:refnum<class "NI_report.lvclass">, "error out"=w1051:errorcluster)  [unwired: 7 in, 3 out]
      n141 = call <vilib>:"Excel Run Macro.vi"("report in"=w1052, "macro name"=w1016, "error in (no error)"=w1051) -> ("report out"=w1050:refnum<class "NI_report.lvclass">, "error out"=w1049:errorcluster)  [unwired: 10 in, 1 out]
      n142 = call <vilib>:"Excel Get Worksheet.vi"("report in"=w1050, "worksheet index (0)"=1, "error in (no error)"=w1049) -> ("report out"=w1047:refnum<class "NI_report.lvclass">, "error out"=w1046:errorcluster)  [unwired: 11 in]
      n143 = call-poly <vilib>:"Append Table to Report.vi"("report in"=w1047, "column headers"=w1019, "text data"="Table Control 2", "error in (no error)"=w1046) -> ("report out"=w1044:refnum<class "NI_report.lvclass">, "error out"=w1043:errorcluster)  [unwired: 8 in, 2 out]
      n144 = call <vilib>:"Excel Insert Cells.vi"("report in"=w1044, "error in (no error)"=w1043) -> ("report out"=w1042:refnum<class "NI_report.lvclass">, "error out"=w1041:errorcluster)  [unwired: 12 in]
      n145 = call <vilib>:"Excel Easy Text.vi"("report in"=w1042, "text"=w1017, "start (-1, -1)"=w1018, "error in (no error)"=w1041) -> ("report out"=w1040:refnum<class "NI_report.lvclass">, "error out"=w1039:errorcluster)  [unwired: 7 in, 3 out]
      n146 = call <vilib>:"Excel Run Macro.vi"("report in"=w1040, "macro name"=w1016, "error in (no error)"=w1039) -> ("report out"=w1038:refnum<class "NI_report.lvclass">, "error out"=w1037:errorcluster)  [unwired: 10 in, 1 out]
      n147 = call <vilib>:"Excel Rename Worksheet.vi"("report in"=w1038, "worksheet name (\"\")"="BGA387" ("worksheet name (\"\")"), "error in (no error)"=w1037) -> ("report out"=w1015:refnum<class "NI_report.lvclass">, "error out"=w1014:errorcluster)  [unwired: 11 in]
      n148 = Format Date/Time String(time format string (%c)="%Y%m%d%H", seconds (now)=w1022) -> (date/time string=w1020:string)  [unwired: 1 in]
      n149 = Concatenate Strings(w1056, w1020, ".xls" ("string")) -> (w1057:string)
      n150 = Concatenate Strings(w1056, w1020) -> ()  [unwired: 1 out]
      n151 = Build Path(base path=path "o:/monitor/report", name or relative path=w1057) -> (appended path=w1055:path)
      n152 = call <vilib>:"Excel Get Worksheet.vi"("report in"=w1015, "worksheet index (0)"=0, "error in (no error)"=w1014) -> ("report out"=w1028:refnum<class "NI_report.lvclass">, "error out"=w1027:errorcluster)  [unwired: 11 in]
      n153 = call-dynamic "Save Report to File.vi"("report in"=w1028, "report file path"=w1055, "error in (no error)"=w1027) -> ("report out"=w1034:refnum<class "NI_report.lvclass">, "error out"=w1033:errorcluster)  [unwired: 11 in]
      n154 = call-dynamic "Dispose Report.vi"("report in"=w1034, "save changes? (F)"=FALSE, "error in (no error)"=w1033) -> ("error out"=→"error out 4":errorcluster)  [unwired: 12 in]
    }
    frame #3 {
      n155 = Index Array(array=w1073) -> (element=w1072:i32)  [unwired: 1 in]
      n156 = Greater?(x=w1072, y=0) -> (0:w1070:bool)
      n157 = case shown="True" w1070 {
        tunnel: w1075 -> [_ w1077]
        tunnel: w1074 -> [_ w1076]
        frame False {
        }
        frame True {
          (unwired) string[] ["yyliao@ptse.com.tw", "E100@ptse.com.tw", "M110@ptse.com.tw", "whlee@ptse.com.tw", "color.yen@mstarsemi.com", "ch.yang@mstarsemi.com", "shang.liang@mstarsemi.com", "hy.chien@mstarsemi.com", "Allonsite@mstarsemi.com", "stanley.wang@mstarsemi.com", "zoe.huang@mstarsemi.com", "doris.lee@mstarsemi.com", "terry.lee@mstarsemi.com", "wj.hung@mstarsemi.com", "frank.liu@mstarsemi.com", "ywcheng@ptse.com.tw", "hzchen@ptse.com.tw", "jcwang@ptse.com.tw", "eric_fan@ptse.com.tw", "saulwang@ptse.com.tw", "jtwu@ptse.com.tw", "sam-cs.lin@mstarsemi.com", "hank.huang@mstarsemi.com", "peggylee@ptse.com.tw", "chialin.wang@mstarsemi.com "] ("recipients")
          (unwired) "***** MStar Special  Monitor  Report from PTS ***" ("subject ([No Subject])")
          n158 = Current VI's Path() -> (path=w1082:path)
          n159 = Strip Path(path=w1082) -> (name=w1081:string)  [unwired: 1 out]
          n160 = Match Pattern(string=w1081, regular expression=".vi") -> (before substring=w1079:string)  [unwired: 1 in, 3 out]
          n161 = call "MailMessage.vi"("AddSubject"=w1076, "message"="如附件", "file path"=w1077, "program"=w1079) -> ()  [unwired: 8 in]
        }
      }
    }
    frame #4 {
      n162 = Quit LabVIEW() -> ()  [unwired: 1 in]
    }
  }
